vi "String Constants.vi"() -> ()   [LabVIEW 2016, in "Scan Engine Custom Device.lvlib"]
uses:
  Scan Engine Custom Device.lvlib
panel:
  in  "DS402 Drive Status Variables":string="Status Information from the Drive"
  in  "DS402 Drive Command Variables":string="Commands to the Drive"
  in  "ECAT I/O Network Variables Output":string="Here the outgoing I/O Network Variable are listed which are hosted on the EtherCAT-Slave."
  in  "ECAT I/O Network Variables Input":string="Here the incoming I/O Network Variable are listed which are hosted on the EtherCAT-Slave."
  in  "Local FPGA Desc":string="A CompactRIO chassis can run a custom FPGA personality created with LabVIEW FPGA. Use this page to import the user variables of the custom personality to NI VeriStand.\n\nUser variable types supported include:\nU32, U16, U8, I32, I16, I8, Boolean, and FXP.\n\nNote: The only supported FXP UDVs are those  with word lengths up to 32 bits, and integer word lengths between -32 and +32."
  in  "AutoDetect Warning":string="This will discover all local and EtherCAT modules currently connected to your system.  However, it will not discover any specific module  settings.  You will need to manually configure your modules after discovery is complete.\n\nThis will also delete your current configuration.\n\nAre you sure you want to continue?"
  in  "Bitfile Scan Modules (2009)":string="/CompilationResults/NiRioScanInterface/CartContSlotInfo/Slot/number/text()"
  in  "Bitfile Scan Modules (2010) - also works":string="/CompilationResults/NiRio/ResourceManager[@name=\"rsiReg_rm\"]/CollectionInfo[@name=\"CartCtrlMemoryRegDeviceCollection\"]/DeviceList/Device/Number/text()"
  in  "Bitfile Scan Modules (2010)":string="/CompilationResults/NiRio/ResourceManager[@name=\"rsiReg_rm\"]/CollectionInfo[@name=\"CartCtrlConfigRegDeviceCollection\"]/DeviceList/Device/Number/text()"
  in  "FXP VI Base Path":path=path "c:/ni-rt/NIVeriStand/Custom Devices/Scan Engine/FXP.llb"
  in  "RT Bitfile Base Path":path=path "c:/ni-rt/NIVeriStand/Custom Devices/Scan Engine/Bitfiles"
  in  "Device Name":string="Scan Engine / EtherCAT"
  in  "ECAT FPGA Desc":string="A NI-9144 EtherCAT chassis can run a custom FPGA personality created with LabVIEW FPGA. After downloading the FPGA personality to the NI-9144 chassis, use this page to import the user variables of the custom personality to NI VeriStand.\n\nUser variable types supported include:\nU32, U16, U8, I32, I16, I8, Boolean, and FXP.\n\nNote: The only supported FXP UDVs are those  with word lengths up to 32 bits, and integer word lengths between -32 and +32."
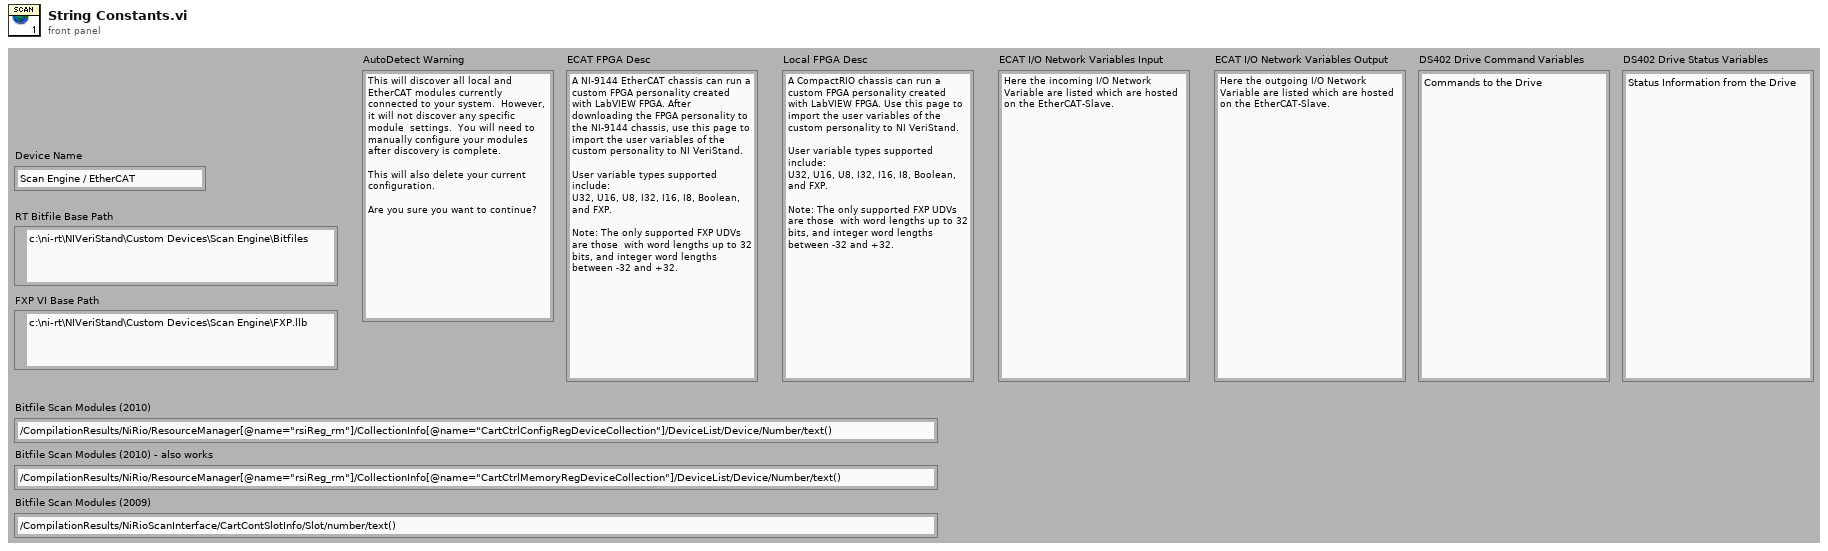
[diagram p1: front panel]
diagram:
